vi "niRFSysCalReader Initialize.vi"(8 "error in":errorcluster, 10 "Path Name":string, 11 "niRFSysCal XML File Path":path) -> (0 "error out":errorcluster, 3 "niRFSysCalReader Handle out":T1)   [LabVIEW 2016, in "niRFSysCalReader.lvlib"]
doc: "Creates a new niRFSysCalReader Handle that stores the calibration data from a NI RF System Calibration XML file into the application's memory."
uses:
  niRFSysCalReader.lvlib
  _INCLUDES/niRFSysCalReader Handle.ctl
  _INCLUDES/niRFSysCalReader Core States.ctl
  <vilib>/Utility/error.llb/Error Cluster From Error Code.vi
  <vilib>/ErrorRing/Error Ring.xnode
  _Dependencies/Pathloss XML Reader/Pathloss XML Reader.lvlib
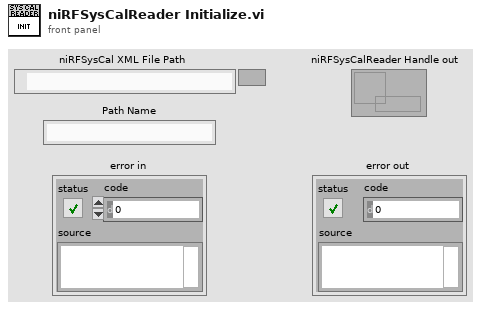
[diagram p1: front panel]
types:
  T1 = typedef "niRFSysCalReader.lvlib/niRFSysCalReader Handle.ctl" = refnum<data-value>
  T2 = typedef "niRFSysCalReader.lvlib/niRFSysCalReader Core States.ctl" = enum16{"Initialize", "Interpolator State", "Add Pathloss", "Get Pathloss", "Remove Pathloss", "Close"}
  T3 = typedef "Pathloss XML Reader.lvlib/XML Reader Data Ref.ctl" = refnum<data-value>
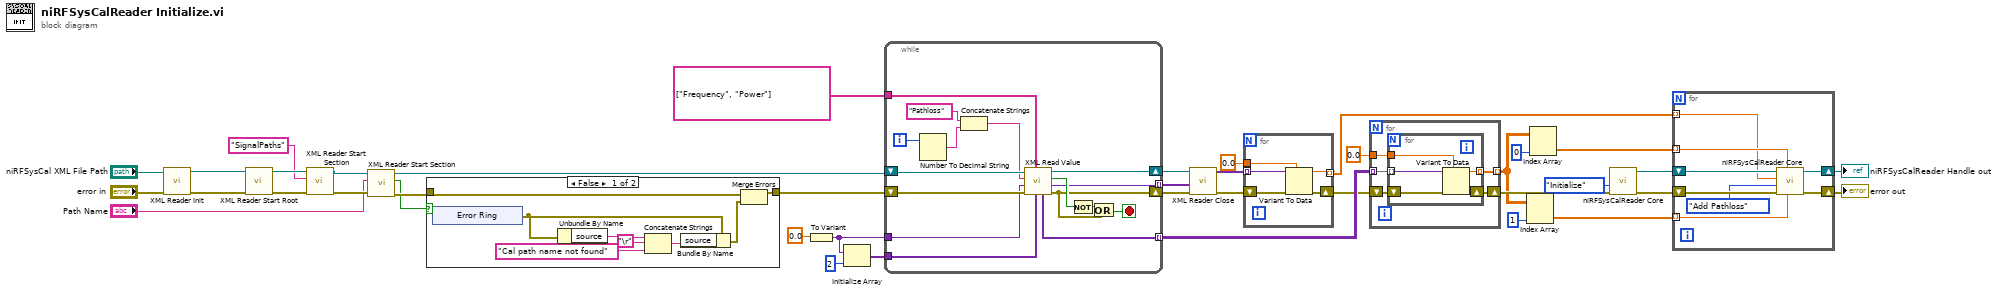
[diagram p0: block diagram]
diagram:
  n1 = call "XML Reader Init.vi"("error in"="error in", "File Path (dialog if empty)"="niRFSysCal XML File Path") -> ("error out"=w35:errorcluster, "XML Reader out"=w39:T3)  [unwired: 8 in]
  n2 = call "XML Reader Start Root.vi"("error in"=w35, "XML Reader In"=w39) -> ("error out"=w34:errorcluster, "XML Reader Out"=w38:T3)  [unwired: 8 in]
  n3 = call "XML Reader Start Section.vi"("error in"=w34, "Element Name"="SignalPaths" ("Section Name"), "XML Reader In"=w38) -> ("error out"=w33:errorcluster, "XML Reader Out"=w32:T3)  [unwired: 5 in, 2 out]
  n4 = call "XML Reader Start Section.vi"("error in"=w33, "Element Name"="Path Name", "XML Reader In"=w32) -> ("error out"=w31:errorcluster, "Found?"=w5:bool, "XML Reader Out"=w20:T3)  [unwired: 5 in, 1 out]
  n5 = case shown="False" w5 {
    tunnel: w31 -> [w46 w52]
    tunnel: [w47 w52] -> w22
    frame False {
      n6 = xnode "Error Ring"() -> ("error out"=w45:errorcluster)
      n7 = Unbundle By Name(w45) -> ("source"=w42:string)
      n8 = Concatenate Strings(w42, "\r", "Cal path name not found" ("error message (\"\")")) -> (w43:string)
      n9 = Bundle By Name(cluster=w45, "source"=w43) -> (w44:errorcluster)
      n10 = Merge Errors(w46, w44) -> (w47:errorcluster)
    }
    frame True {
    }
  }
  n11 = To Variant(anything=0.0 ("Default Element Value")) -> (Variant=w16:variant)
  n12 = Initialize Array(w16, 2 ("dimension size")) -> (w17:variant[])
  n13 = while {
    tunnel: w16 -> [w61]
    tunnel: [w57] -> w29 mode=indexing
    tunnel: string[] ["Frequency", "Power"] ("Attribute Names") -> [w55]
    tunnel: w17 -> [w54]
    tunnel: [w53] -> w26 mode=indexing
    shift-right: [w59] -> w28
    shift-left: w22 -> [w67]
    shift-right: [w66] -> w30
    shift-left: w20 -> [w68]
    i -> [w65]
    stop <- w58 stop-if-true
    n14 = Number To Decimal String(number=w65) -> (decimal integer string=w63:string)  [unwired: 1 in]
    n15 = Concatenate Strings("Pathloss" ("string"), w63) -> (w62:string)
    n16 = call "XML Read Value.vi"("Default Attribute Values"=w54, "Attribute Names"=w55, "error in (no error)"=w67, "Default Element Value"=w61, "Element Name"=w62, "XML Reader In"=w68) -> ("error out"=w59:errorcluster, "Element Value"=w57:variant, "Found?"=w60:bool, "XML Reader Out"=w66:T3, "Attribute Values"=w53:variant[])  [unwired: 1 in]
    n17 = Not(x=w60) -> (.not. x?=w56:bool)
    n18 = Or(x=w56, y=w59) -> (x .or. y?=w58:bool)
  }
  n19 = call "XML Reader Close.vi"("error in"=w28, "XML Reader In"=w30) -> ("error out"=w27:errorcluster)  [unwired: 9 in]
  n20 = for {
    tunnel: w29 -> [w73] mode=indexing
    tunnel: 0.0 ("Default Element Value") -> [w72]
    tunnel: [w70] -> w1 mode=indexing
    shift-right: [w69] -> w25
    shift-left: w27 -> [w71]
    n21 = Variant To Data(error in=w71, type=w72, Variant=w73) -> (data=w70:dbl, error out=w69:errorcluster)
  }
  n22 = for {
    tunnel: w26 -> [w78] mode=indexing
    tunnel: [w76] -> w2 mode=indexing
    shift-right: [w75] -> w12
    shift-left: w25 -> [w77]
    tunnel: 0.0 ("Default Element Value") -> [w74]
    n23 = for {
      tunnel: w78 -> [w83] mode=indexing
      tunnel: [w81] -> w76 mode=indexing
      tunnel: w74 -> [w79]
      shift-right: [w80] -> w75
      shift-left: w77 -> [w82]
      n24 = Variant To Data(error in=w82, type=w79, Variant=w83) -> (data=w81:dbl, error out=w80:errorcluster)
    }
  }
  n25 = Index Array(array=w2, index (col)=1 ("disabled index (col)")) -> (element=w10:dbl[])  [unwired: 1 in]
  n26 = Index Array(array=w2, index (col)=0 ("disabled index (col)")) -> (element=w8:dbl[])  [unwired: 1 in]
  n27 = call "niRFSysCalReader Core.vi"("error in"=w12, "niRFSysCalReader State"=niRFSysCalReader_Core_States."Initialize" ("Cal Storage")) -> ("error out"=w11:errorcluster, "niRFSysCalReader Handle out"=w7:T1)  [unwired: 7 in, 1 out]
  n28 = for {
    shift-right: [w91] -> w4
    shift-left: w11 -> [w90]
    tunnel: w10 -> [w89] mode=indexing
    tunnel: w8 -> [w88] mode=indexing
    tunnel: w1 -> [w86] mode=indexing
    shift-right: [w85] -> w3
    shift-left: w7 -> [w87]
    n29 = call "niRFSysCalReader Core.vi"("Power (dBm)"=w89, "Frequency (Hz)"=w88, "error in"=w90, "niRFSysCalReader State"=niRFSysCalReader_Core_States."Add Pathloss" ("Cal Storage"), "Pathloss (dB)"=w86, "niRFSysCalReader Handle"=w87) -> ("error out"=w91:errorcluster, "niRFSysCalReader Handle out"=w85:T1)  [unwired: 3 in, 1 out]
  }
  "niRFSysCalReader Handle out" <- w3
  "error out" <- w4
